vi "svc_Value to Histogram Bin Index.vi"(7 "evenly spaced (F)":bool, 10 "value":dbl=10.0, 11 "bins in":T1[](array[typedef]) {"upper" format="%0.2f"; "lower" format="%0.2f"}) -> (2 "bin index":i32, 3 "bins out":T1[](array[typedef]) {"upper" format="%0.2f"; "lower" format="%0.2f"})   [LabVIEW 2017]
uses:
  <vilib>/addons/_NISVFA/_Shared subVIs/Controls/svc_Bin Specification.ctl
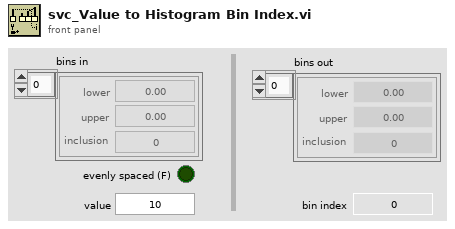
[diagram p1: front panel]
types:
  T1 = typedef "svc_Bin Specification.ctl" = cluster{"lower":dbl, "upper":dbl, "inclusion":u32}
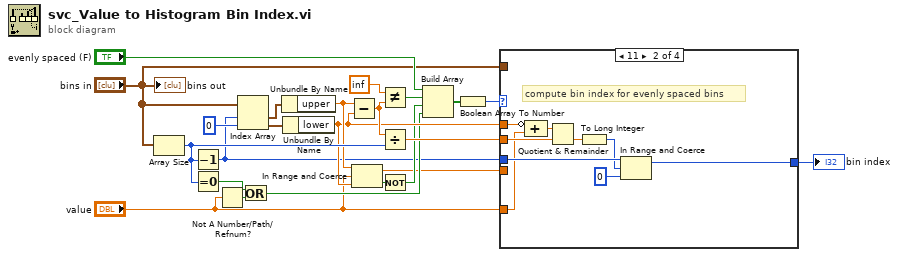
[diagram p0: block diagram]
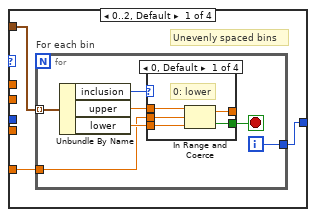
[diagram p2: hidden frame]
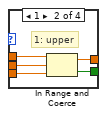
[diagram p3: hidden frame]
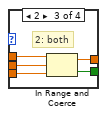
[diagram p4: hidden frame]
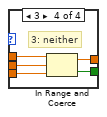
[diagram p5: hidden frame]
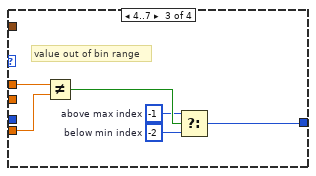
[diagram p6: hidden frame]
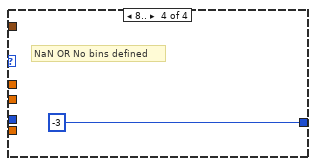
[diagram p7: hidden frame]
diagram:
  n1 = Array Size(array="bins in") -> (size(s)=w15:i32)
  n2 = Decrement(x=w15) -> (x-1=w4:i32)
  n3 = Equal To 0?(x=w15) -> (x = 0?=w22:bool)
  n4 = Not A Number/Path/Refnum?(number/path/refnum="value") -> (NaN/Path/Refnum?=w23:bool)
  n5 = Index Array(array="bins in", index #1=w4, index #2=0 ("index")) -> (element #1=w21:T1, element #2=w19:T1)
  n6 = Or(x=w22, y=w23) -> (x .or. y?=w8:bool)
  n7 = Unbundle By Name(w21) -> ("upper"=w14:dbl)
  n8 = Unbundle By Name(w19) -> ("lower"=w13:dbl)
  n9 = Subtract(x=w14, y=w13) -> (x-y=w17:dbl)
  n10 = In Range and Coerce(upper limit=w14, x="value", lower limit=w13) -> (coerced(x)=w2:dbl, In Range?=w7:bool)
  n11 = Not Equal?(x=inf, y=w17) -> (x != y?=w12:bool)
  n12 = Divide(x=w17, y=w15) -> (x/y=w16:dbl)
  n13 = Not(x=w7) -> (.not. x?=w6:bool)
  n14 = Build Array("evenly spaced (F)", w12, w6, w8) -> (w10:bool[])
  n15 = Boolean Array To Number(Boolean array=w10) -> (number=w9:u32)
  n16 = case shown="11" w9 {
    tunnel: w13 -> [_ w62 w64 _]
    tunnel: w16 -> [_ w60 _ _]
    tunnel: w4 -> [_ w58 _ _]
    tunnel: [w24 w55 w63 -3 ("f")] -> w1
    tunnel: "bins in" -> [w26 _ _ _]
    tunnel: "value" -> [w25 w54 _ _]
    tunnel: w2 -> [_ _ w65 _]
    frame 0..2, Default {
      # "Unevenly spaced bins"
      n17 = for "For each bin" {
        tunnel: w26 -> [w28] mode=indexing
        tunnel: w25 -> [w32]
        tunnel: [w29] -> w24
        i -> [w29]
        stop <- w27 stop-if-true
        n18 = Unbundle By Name(w28) -> ("inclusion"=w30:u32, "upper"=w31:dbl, "lower"=w33:dbl)
        n19 = case shown="0, Default" w30 {
          tunnel: w31 -> [w38 w43 w48 w53]
          tunnel: w33 -> [w37 w42 w47 w52]
          tunnel: w32 -> [w36 w41 w46 w51]
          tunnel: [w35 w40 w45 w50] -> w27
          tunnel: [w34 w39 w44 w49] -> _
          frame 0, Default {
            # "0: lower"
            n20 = In Range and Coerce(upper limit=w38, x=w36, lower limit=w37) -> (coerced(x)=w34:dbl, In Range?=w35:bool)
          }
          frame 1 {
            # "1: upper"
            n21 = In Range and Coerce(upper limit=w43, x=w41, lower limit=w42) -> (coerced(x)=w39:dbl, In Range?=w40:bool)
          }
          frame 2 {
            # "2: both"
            n22 = In Range and Coerce(upper limit=w48, x=w46, lower limit=w47) -> (coerced(x)=w44:dbl, In Range?=w45:bool)
          }
          frame 3 {
            # "3: neither"
            n23 = In Range and Coerce(upper limit=w53, x=w51, lower limit=w52) -> (coerced(x)=w49:dbl, In Range?=w50:bool)
          }
        }
      }
    }
    frame 3 {
      # "compute bin index for evenly spaced bins"
      n24 = Compound Arithmetic op=ADD(invert w62, w54) -> (w61:dbl)
      n25 = Quotient & Remainder(x=w61, y=w60) -> (floor(x/y)=w59:dbl)  [unwired: 1 out]
      n26 = To Long Integer(number=w59) -> (32bit integer=w56:i32)
      n27 = In Range and Coerce(upper limit=w58, x=w56, lower limit=0) -> (coerced(x)=w55:i32)  [unwired: 1 out]
    }
    frame 4..7 {
      w67 = -2  # below min index
      w66 = -1  # above max index
      # "value out of bin range"
      n28 = Not Equal?(x=w64, y=w65) -> (x != y?=w68:bool)
      n29 = Select(t=w66, s=w68, f=w67) -> (s? t:f=w63:i32)
    }
    frame 8.. {
      # "NaN OR No bins defined"
    }
  }
  "bin index" <- w1
  "bins out" <- "bins in"
